vi "Celsius to Fahrenheit Local Variables.vi"() -> ()   [LabVIEW 2023]
panel:
  out "Celsius Temp":dbl(slide) scale=0.0..1000.0
  out "Fahrenheit Temp":dbl(slide) scale=0.0..2000.0
  in  "stop":bool
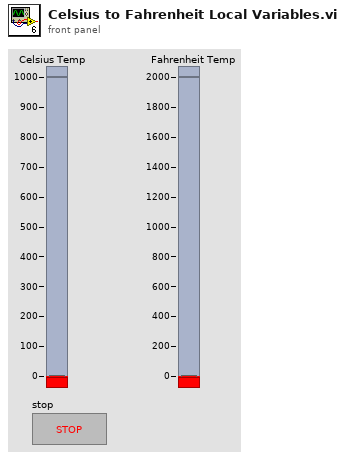
[diagram p1: front panel]
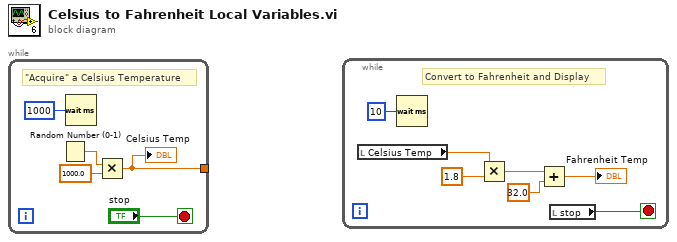
[diagram p0: block diagram]
diagram:
  n1 = while {
    tunnel: [w1] -> _
    stop <- "stop" stop-if-true
    # "\"Acquire\" a Celsius Temperature"
    n2 = Random Number (0-1)() -> (number: 0 to 1=w5:dbl)
    n3 = Wait (ms)(milliseconds to wait=u32 1000) -> ()  [unwired: 1 out]
    n4 = Multiply(x=w5, y=1000.0) -> (x*y=w1:dbl)
    "Celsius Temp" <- w1
  }
  n5 = while {
    stop <- w6 stop-if-true
    # "Convert to Fahrenheit and Display"
    n6 = local read "Celsius Temp"() -> (w7:dbl)
    n7 = Wait (ms)(milliseconds to wait=u32 10) -> ()  [unwired: 1 out]
    n8 = Multiply(x=w7, y=1.8) -> (x*y=w11:dbl)
    n9 = Add(x=w11, y=32.0) -> (x+y=→"Fahrenheit Temp":dbl)
    n10 = local read "stop"() -> (w6:bool)
  }
